vi "read channels of classification.vi"(6 "channel classification":T2, 8 "error in":errorcluster, 11 "Shared Memory runtime in":refnum<class "Shared Memory runtime.lvclass">) -> (0 "error out":errorcluster, 2 "channels":T1[](array[typedef]), 3 "Shared Memory runtime out":refnum<class "Shared Memory runtime.lvclass">)   [LabVIEW 2013, in "Shared Memory runtime.lvclass"]
uses:
  Shared Memory runtime.lvclass
  <vilib>/NI/Tag Bus Module Framework/channel/channel classification.ctl
  channel runtime.ctl
  <vilib>/NI/Tag Bus/tag/Data Type.ctl
  <vilib>/National Instruments/Shared Memory Library for Linux RT/Controls/Shared Memory Class Reference.ctl
  <vilib>/National Instruments/Shared Memory Library for Linux RT/Classes/Shared Memory/Shared Memory.lvclass
  Shared Memory runtime.lvclass/Shared Memory runtime.ctl
  Read input data.vi
  Read processing parameter.vi
  Read processing results.vi
  Read output data.vi
  <vilib>/NI/Tag Bus Module Framework/channel/TBM channel.lvclass
  <vilib>/NI/Tag Bus/tag/tag descriptor.lvclass
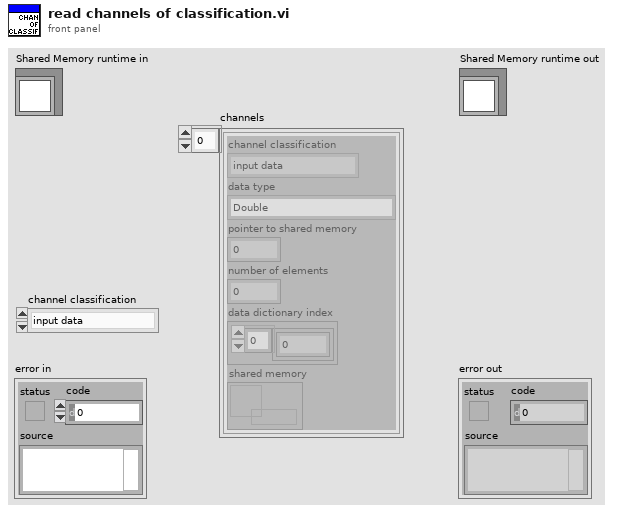
[diagram p1: front panel]
types:
  T1 = typedef "Shared Memory runtime.lvclass/channel runtime.ctl" = cluster{"channel classification":T2, "data type":T3, "pointer to shared memory":u64, "number of elements":u64, "data dictionary index":cluster{i32[]}, "shared memory":T4}
  T2 = typedef "TBM channel.lvclass/channel classification.ctl" = enum16{"input data", "output data", "processing parameter", "processing result"}
  T3 = typedef "tag bus.lvlib/tag descriptor.lvclass/Data Type.ctl" = enum16{"Double", "Single", "I64", "I32", "I16", "I8", "U64", "U32", "U16", "U8", "Boolean", "String", "Array of Double", "Array of Single", "Array of I64", "Array of I32", "Array of I16", "Array of I8", "Array of U64", "Array of U32", "Array of U16", "Array of U8", "Array of Boolean", "Array of String"}
  T4 = typedef "Shared Memory Class Reference.ctl" = refnum<data-value>
  T5 = cluster{"channel classification":T2, "data type":T3, "pointer to shared memory":u64, "number of elements":u64, "data dictionary index":cluster{i32[]}, "shared memory":T4}[]
  T6 = cluster{"channel classification":T2, "data type":T3, "pointer to shared memory":u64, "number of elements":u64, "data dictionary index":cluster{i32[]}, "shared memory":T4}[][]
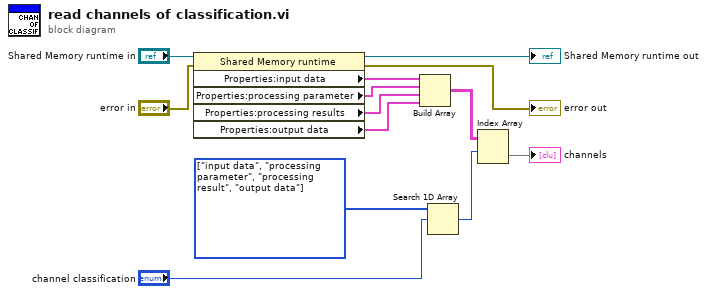
[diagram p0: block diagram]
diagram:
  w10 = T2[] [enum."input data", enum."processing parameter", enum."processing result", enum."output data"] items=["input data", "output data", "processing parameter", "processing result"] ("supported classifications")
  n1 = property class="Shared Memory runtime"(reference="Shared Memory runtime in", error in="error in") -> (reference out=→"Shared Memory runtime out":refnum<class "Shared Memory runtime.lvclass">, error out=→"error out":errorcluster, "Properties:input data"=w13:T5, "Properties:processing parameter"=w9:T5, "Properties:processing results"=w8:T5, "Properties:output data"=w7:T5)
  n2 = Build Array(w13, w9, w8, w7) -> (w11:T6)
  n3 = Search 1D Array(1D array=w10, element="channel classification") -> (index of element=w12:i32)  [unwired: 1 in]
  n4 = Index Array(array=w11, index (row)=w12) -> (element=→"channels":T5)  [unwired: 1 in]
